vi "C(T) data acquisition loop.vi"(0 "Path in":path, 5 "Temp Array In":dbl[](array[numeric]) format="%.2f", 7 "Timing Control Parameters In":T1={"N cycles for averaging"=100, "N points per measurement"=1000, "Measurment time interval"=1e-05} {"Measurment time interval" format="%.2e"}, 11 "error in":errorcluster) -> (4 "Path out":path, 6 "Temp Array Out":dbl[](array[numeric]) format="%.2f", 8 "Timing Control Parameters Out":T1={"N cycles for averaging"=100, "N points per measurement"=1000, "Measurment time interval"=1e-05} {"Measurment time interval" format="%.2e"}, 10 "Normalized Data Out":waveform(dbl)[](array[waveform]), 15 "error out":errorcluster)   [LabVIEW 2014]
doc: "this subvi manages the capacitance measurement cycle\n\nPaul K Dixon\nPhysics 350\nCSUSB Physics"
uses:
  globals/C(T) global variables.vi
panel:
  # "C(T) Acquisition Loop"
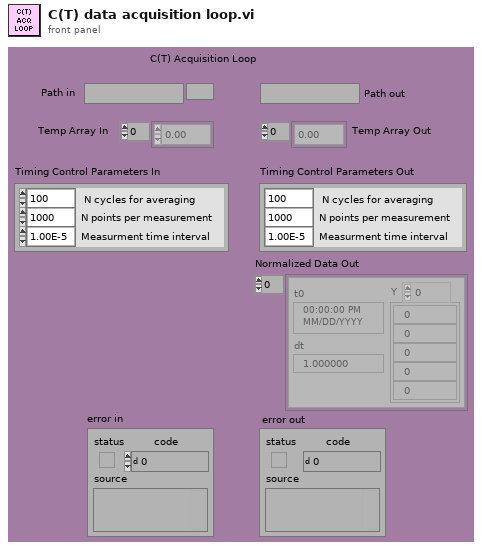
[diagram p1: front panel]
types:
  T1 = cluster{"N cycles for averaging":i32, "N points per measurement":i32, "Measurment time interval":dbl}
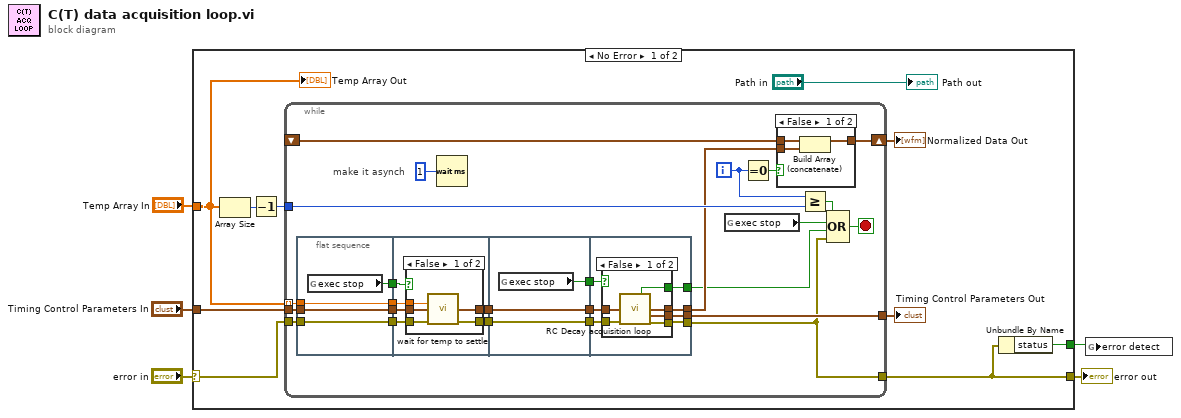
[diagram p0: block diagram]
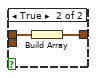
[diagram p4: hidden frame]
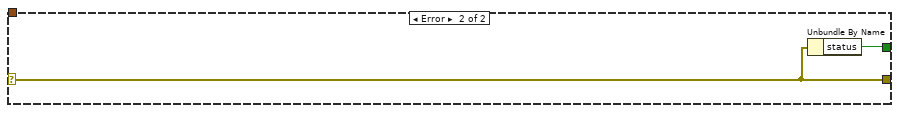
[diagram p5: hidden frame]
diagram:
  n1 = case shown="No Error" "error in" {
    selector: "error in" -> [w8 w82]
    tunnel: "Timing Control Parameters In" -> [w12 _]
    tunnel: [w7 w82] -> w3
    tunnel: "Temp Array In" -> [w9 _]
    tunnel: [w6 w81] -> w1
    frame No Error {
      n2 = Array Size(array=w9) -> (size(s)=w15:i32)
      n3 = Decrement(x=w15) -> (x-1=w14:i32)
      n4 = while {
        tunnel: [w20] -> w11
        shift-left: _ -> [w36]
        shift-right: [w39] -> w13
        tunnel: w14 -> [w40]
        tunnel: w9 -> [w25] mode=indexing
        tunnel: w12 -> [w24]
        tunnel: w8 -> [w18]
        tunnel: [w16] -> w7
        i -> [w38]
        stop <- w33 stop-if-true
        # "make it asynch"
        n5 = flat-sequence {
          tunnel: [w44] -> w31
          tunnel: w25 -> [w43]
          tunnel: w24 -> [w42]
          tunnel: [w43] -> w23
          tunnel: [w42] -> w22
          tunnel: w18 -> [w41]
          tunnel: [w41] -> w17
          tunnel: w31 -> [w50]
          tunnel: [w49] -> w30
          tunnel: [w45] -> w29
          tunnel: w23 -> [w48]
          tunnel: w22 -> [w47]
          tunnel: w17 -> [w46]
          tunnel: [w60] -> w28
          tunnel: w30 -> [w60]
          tunnel: [w59] -> w27
          tunnel: w29 -> [w59]
          tunnel: [w58] -> w26
          tunnel: w28 -> [w67]
          tunnel: w27 -> [w66]
          tunnel: w26 -> [w65]
          tunnel: [w64] -> w21
          tunnel: [w63] -> w20
          tunnel: [w62] -> w16
          tunnel: [w61] -> w19
          frame #0 {
            n6 = global read "C(T) global variables.vi" "exec stop"() -> (w44:bool)
          }
          frame #1 {
            n7 = case shown="False" w50 {
              tunnel: [w54 w57] -> w49
              tunnel: w48 -> [w53 _]
              tunnel: w47 -> [w52 w57]
              tunnel: w46 -> [w51 w56]
              tunnel: [w55 w56] -> w45
              frame False {
                n8 = call "wait for temp to settle.vi"("Current setpoint"=w53, "Timing Control Parameters In"=w52, "error in"=w51) -> ("Timing Control Parameters Out"=w54:T1, "error out"=w55:errorcluster)  [unwired: 2 in, 9 out]
              }
              frame True {
              }
            }
          }
          frame #2 {
            n9 = global read "C(T) global variables.vi" "exec stop"() -> (w58:bool)
          }
          frame #3 {
            n10 = case shown="False" w65 {
              tunnel: [w73 _] -> w61
              tunnel: [w72 w75] -> w62
              tunnel: [w71 _] -> w64
              tunnel: [w70 w74] -> w63
              tunnel: w66 -> [w69 w75]
              tunnel: w67 -> [w68 w74]
              frame False {
                n11 = call "RC Decay acquisition loop.vi"("Timing Control Parameters In"=w68, "error in (no error)"=w69) -> ("time-out?"=w73:bool, "Normalized Waveform Out"=w71:waveform(dbl), "Timing Control Parameters Out"=w70:T1, "error out"=w72:errorcluster)  [unwired: 10 out]
              }
              frame True {
              }
            }
          }
        }
        n12 = Wait (ms)(milliseconds to wait=u32 1) -> ()  [unwired: 1 out]
        n13 = global read "C(T) global variables.vi" "exec stop"() -> (w32:bool)
        n14 = Equal To 0?(x=w38) -> (x = 0?=w37:bool)
        n15 = case shown="False" w37 {
          tunnel: w21 -> [w76 w80]
          tunnel: [w77 w79] -> w39
          tunnel: w36 -> [w78 _]
          frame False {
            n16 = Build Array (concatenate)(w78, w76) -> (w77:waveform(dbl)[])
          }
          frame True {
            n17 = Build Array(w80) -> (w79:waveform(dbl)[])
          }
        }
        n18 = Greater Or Equal?(x=w38, y=w40) -> (x >= y?=w34:bool)
        n19 = Compound Arithmetic op=OR(w34, w32, w19, w16) -> (w33:bool)
      }
      "Normalized Data Out" <- w13
      "Timing Control Parameters Out" <- w11
      n20 = Unbundle By Name(w7) -> ("status"=w6:bool)
      "Temp Array Out" <- w9
      "Path out" <- "Path in"
    }
    frame Error {
      n21 = Unbundle By Name(w82) -> ("status"=w81:bool)
    }
  }
  "error out" <- w3
  n22 = global write "C(T) global variables.vi" "error detect"(w1) -> ()
